vi "Motic Set Binning Index.vi"(8 "error in (no error)":errorcluster, 10 "idx":i32, 11 "camera":i32) -> (0 "error out":errorcluster, 3 "camera out":i32)   [LabVIEW 2012, in "MoticApi.lvlib"]
doc: "MOTICAPI bool Motic_setBinningIndex(MUCam_Handle camera, int idx);"
uses:
  MoticApi.lvlib
  MoticApi.dll
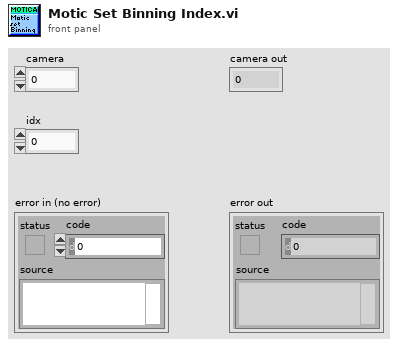
[diagram p1: front panel]
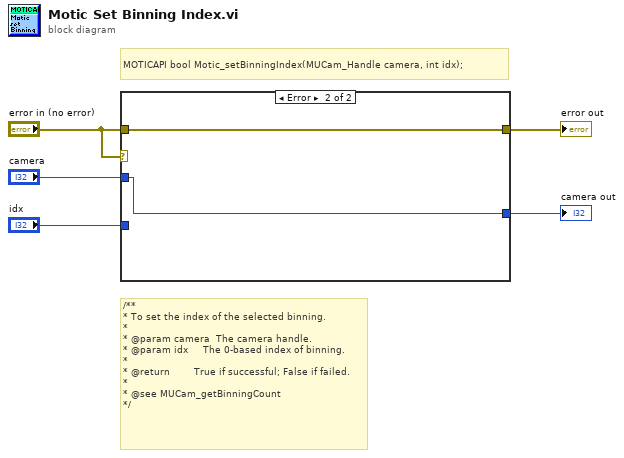
[diagram p0: block diagram]
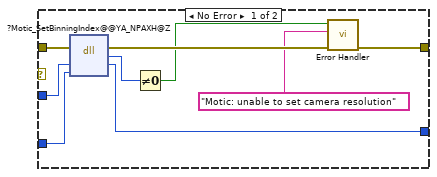
[diagram p2: hidden frame]
diagram:
  # "/**\n* To set the index of the selected binning.\n*\n* @param camera  The camera handle.\n* @param idx     The 0-based index of binning.\n*\n* @return        True if successful; False if failed.\n*\n* @see MUCam_getBinningCount\n*/"
  # "MOTICAPI bool Motic_setBinningIndex(MUCam_Handle camera, int idx);"
  n1 = case shown="Error" "error in (no error)" {
    tunnel: "camera" -> [w13 w15]
    tunnel: [w12 w15] -> w4
    tunnel: "idx" -> [w11 _]
    tunnel: "error in (no error)" -> [w10 w16]
    tunnel: [w8 w16] -> w2
    frame No Error {
      n2 = dll-call lib="C:/Users/TTS-Digital/Desktop/MoticApi/MoticApi_git/MoticApi/MoticApi.*" fn="?Motic_SetBinningIndex@@YA_NPAXH@Z"(error in=w10, "camera"=w13, "idx"=w11) -> (error out=w9:errorcluster, "return type"=w14:u8, "camera"=w12:i32)  [unwired: 3 in, 1 out]
      n3 = Not Equal To 0?(x=w14) -> (x != 0?=w7:bool)
      n4 = call "Error Handler.vi"("error in (no error)"=w9, "Error message"="Motic: unable to set camera resolution" ("source"), "Function return"=w7) -> ("error out"=w8:errorcluster)  [unwired: 8 in]
    }
    frame Error {
    }
  }
  "camera out" <- w4
  "error out" <- w2
